vi "publishJobStarted.vi"(8 "error in (no error)":errorcluster, 11 "Job in":refnum<class "Job.lvclass">) -> (0 "error out":errorcluster, 3 "Job out":refnum<class "Job.lvclass">)   [LabVIEW 2013, in "openCronJob.lvlib" / "Job.lvclass"]
uses:
  Job.lvclass
  Job Started -- cluster.ctl
  Job.lvclass/Job.ctl
  JobReport/JobReport.lvclass
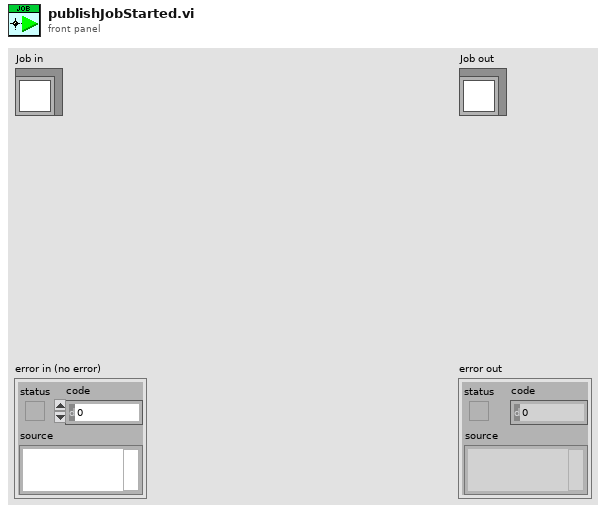
[diagram p1: front panel]
types:
  T1 = typedef "openCronJob.lvlib/Job.lvclass/Job Started -- cluster.ctl" = cluster{"Name":string, "GUID":string, "Time Stamp":timestamp}
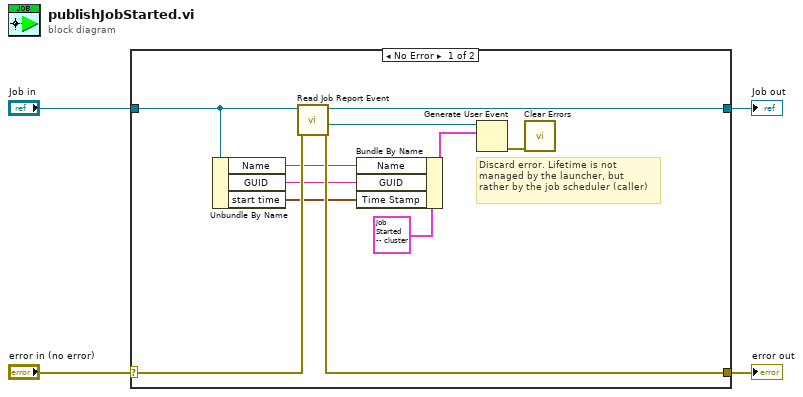
[diagram p0: block diagram]
diagram:
  n1 = case shown="No Error" "error in (no error)" {
    selector: "error in (no error)" -> [w14 w17]
    tunnel: [w13 w17] -> w3
    tunnel: [w15 w16] -> w1
    tunnel: "Job in" -> [w8 w16]
    frame No Error {
      # "Discard error. Lifetime is not\nmanaged by the launcher, but\nrather by the job scheduler (caller)"
      n2 = Unbundle By Name(w8) -> ("Name"=w7:string, "GUID"=w6:string, "start time"=w5:timestamp)
      n3 = call "Read Job Report Event.vi"("error in (no error)"=w14, "Job in"=w8) -> ("error out"=w13:errorcluster, "Job Started Event"=w12:refnum<user-event>, "Job out"=w15:refnum<class "Job.lvclass">)  [unwired: 6 in, 1 out]
      n4 = Bundle By Name(cluster=T1 {"Name"="", "GUID"="", "Time Stamp"=timestamp(0 s since 1904-01-01)} ("Job Started"), "Name"=w7, "GUID"=w6, "Time Stamp"=w5) -> (w9:T1)
      n5 = Generate User Event(user event=w12, event data cluster=w9) -> (error out=w11:errorcluster)  [unwired: 2 in, 1 out]
      n6 = call <vilib>:"Clear Errors.vi"("error in (no error)"=w11) -> ()  [unwired: 6 in, 1 out]
    }
    frame Error {
    }
  }
  "error out" <- w3
  "Job out" <- w1
